vi "db.vi"() -> ()   [LabVIEW 2016]
panel:
  in  "OK Button":bool
  out "Data 2":string[][](array[string])
  in  "stop":bool
  out "Data":string[][](array[string])
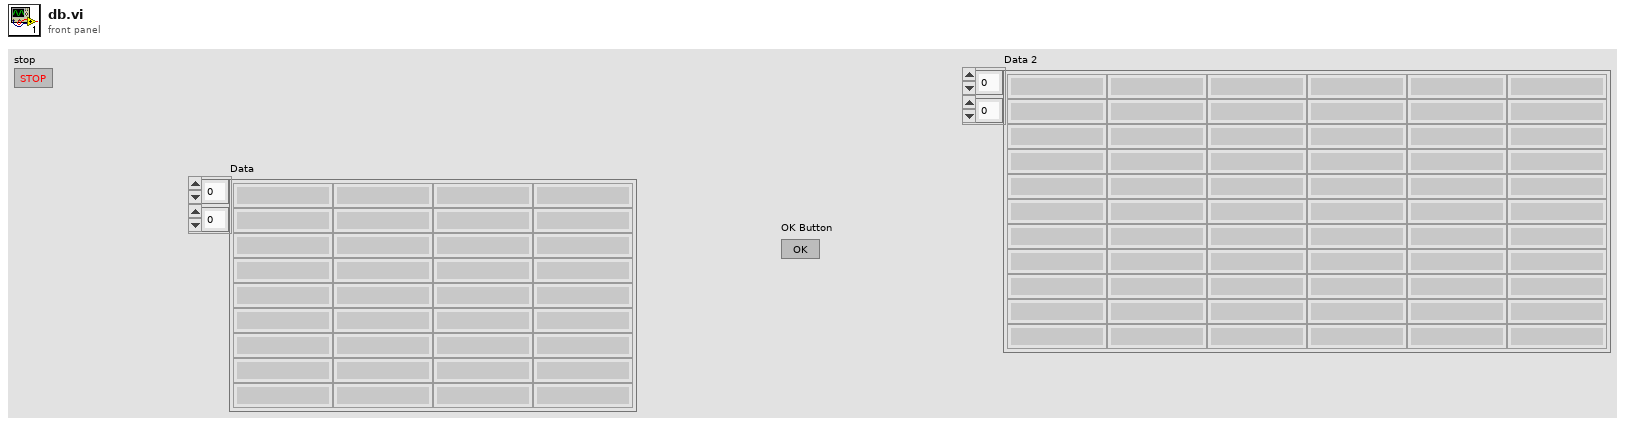
[diagram p1: front panel]
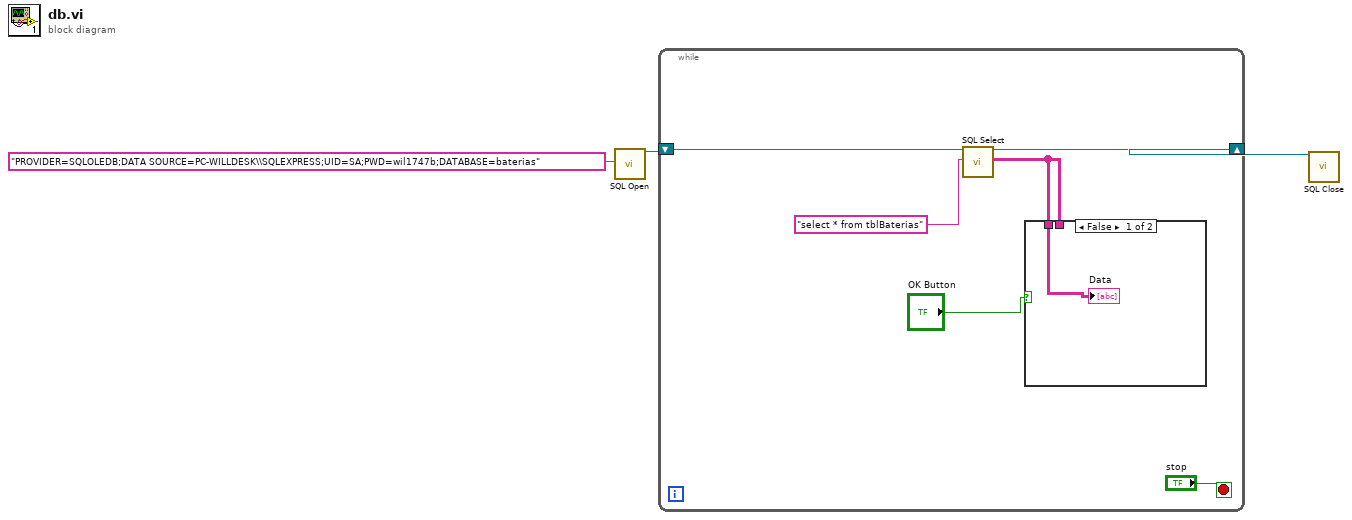
[diagram p0: block diagram]
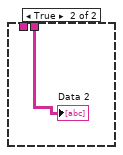
[diagram p2: hidden frame]
diagram:
  n1 = call <vilib>:"SQL Open.vi"("ConnectionString In"="PROVIDER=SQLOLEDB;DATA SOURCE=PC-WILLDESK\\SQLEXPRESS;UID=SA;PWD=wil1747b;DATABASE=baterias") -> ("Connection Out"=w3:refnum<k7>)  [unwired: 17 in, 1 out]
  n2 = while {
    shift-right: [w8] -> w2
    shift-left: w3 -> [w7]
    stop <- "stop" stop-if-true
    n3 = call <vilib>:"SQL Select.vi"("Connection In"=w7, "SQL Query"="select * from tblBaterias") -> ("Connection Out"=w8:refnum<k7>, "Data"=w6:string[][])  [unwired: 15 in, 1 out]
    n4 = case shown="False" "OK Button" {
      tunnel: w6 -> [_ w11]
      tunnel: w6 -> [w10 _]
      frame False {
        "Data" <- w10
      }
      frame True {
        "Data 2" <- w11
      }
    }
  }
  n5 = call <vilib>:"SQL Close.vi"("Connection In"=w2) -> ()  [unwired: 18 in, 1 out]
